vi "FindTestClasses.vi"(8 "error in (no error)":errorcluster, 11 "repository file path":path) -> (0 "error out":errorcluster, 3 "Test Classes":path[](array[path]))   [LabVIEW 2027, in "DiscoverTestCases.lvclass"]
uses:
  DiscoverTestCases.lvclass
  <vilib>/addons/_JKI Toolkits/VI Tester/TestCase.llb/TestCase.lvclass
  DiscoverTestCases.lvclass/DiscoverTestCases.ctl
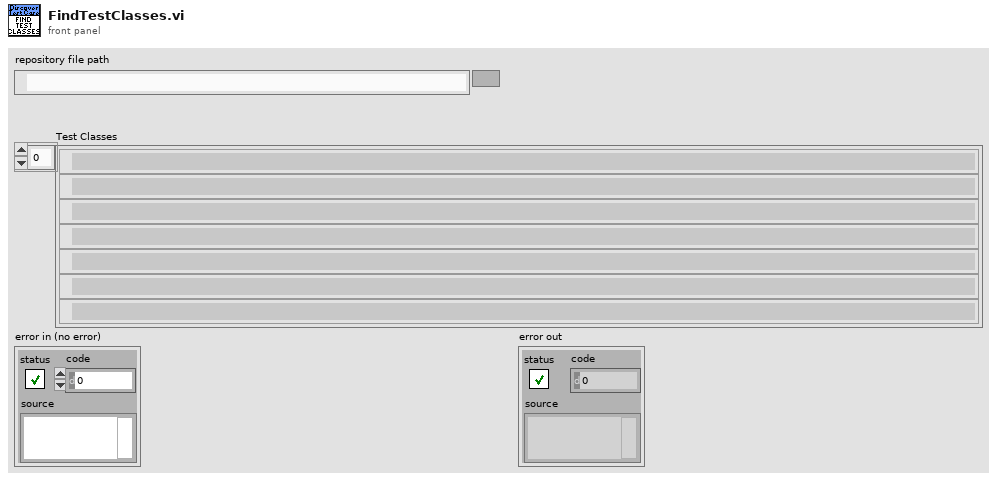
[diagram p1: front panel]
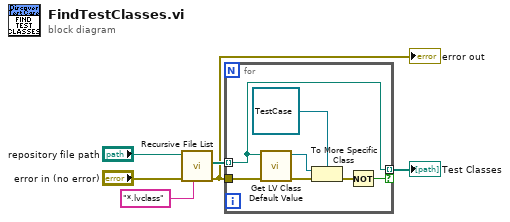
[diagram p0: block diagram]
diagram:
  n1 = call <vilib>:"Recursive File List.vi"("pattern"="*.lvclass", "error in (no error)"="error in (no error)", "Folder Path"="repository file path") -> ("error out"=w2:errorcluster, "All Files in Dir"=w4:path[])  [unwired: 4 in, 3 out]
  "error out" <- w2
  n2 = for {
    tunnel: w4 -> [w11] mode=indexing
    tunnel: [w11] -> w3 mode=indexing if=w9
    tunnel: w2 -> [w8]
    n3 = call <vilib>:"Get LV Class Default Value.vi"("error in (no error)"=w8, "class path"=w11) -> ("error out"=w13:errorcluster, "object"=w12:refnum<class>)  [unwired: 8 in]
    n4 = To More Specific Class(target class=refnum<class "TestCase.lvclass"> refnum ("TestCase in"), reference=w12, error in=w13) -> (error out=w10:errorcluster)  [unwired: 1 out]
    n5 = Not(x=w10) -> (.not. x?=w9:bool)
  }
  "Test Classes" <- w3
